vi "Launch Nested Actor with Map.vi"(8 "error in (no error)":errorcluster, 11 "Calling Actor in":refnum<class "Calling Actor.lvclass">) -> (0 "error out":errorcluster, 3 "Calling Actor out":refnum<class "Calling Actor.lvclass">)   [LabVIEW 2019, in "Calling Actor.lvlib" / "Calling Actor.lvclass"]
uses:
  Calling Actor.lvclass
  C:/Program Files (x86)/National Instruments/LabVIEW 2019/vi.lib/ActorFramework/Actor/Actor.lvclass
  Nested Actor/Nested Actor.lvclass
  Calling Actor.lvclass/Calling Actor.ctl
  <vilib>/ActorFramework/Actor/Actor.lvclass
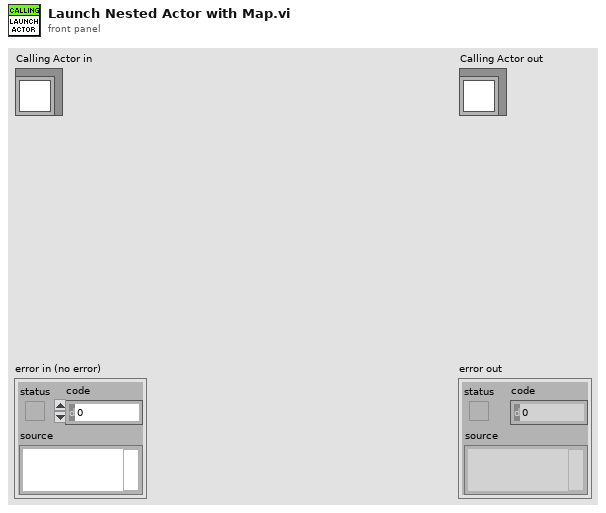
[diagram p1: front panel]
types:
  T1 = map{string, refnum<class "Message Enqueuer.lvclass">}
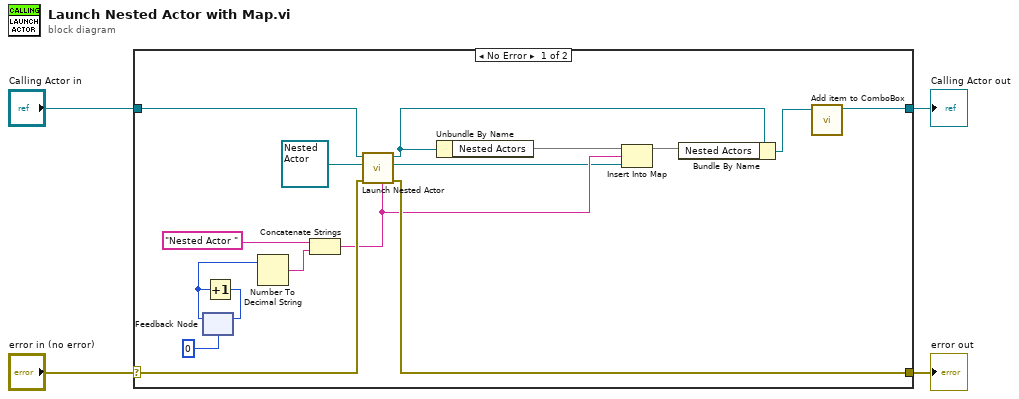
[diagram p0: block diagram]
diagram:
  n1 = case shown="No Error" "error in (no error)" {
    selector: "error in (no error)" -> [w19 w22]
    tunnel: [w18 w22] -> w3
    tunnel: [w11 w21] -> w1
    tunnel: "Calling Actor in" -> [w20 w21]
    frame No Error {
      n2 = feedback #1(0) -> (w14:i32)
      n3 = Increment(x=w14) -> (x+1=w15:i32)
      n4 = feedback-in #1(w15) -> ()
      n5 = Number To Decimal String(number=w14) -> (decimal integer string=w13:string)  [unwired: 1 in]
      n6 = Concatenate Strings("Nested Actor ", w13) -> (w9:string)
      n7 = call <vilib>:"Launch Nested Actor.vi"("Debug Alias"=w9, "error in (no error)"=w19, "Nested Actor"=refnum<class "Nested Actor.lvclass"> refnum ("Nested Actor.lvlib:Nested Actor.lvclass"), "Caller Actor in"=w20) -> ("error out"=w18:errorcluster, "Nested Actor's Enqueuer"=w8:refnum<class "Message Enqueuer.lvclass">, "Caller Actor out"=w7:refnum<class "Calling Actor.lvclass">)  [unwired: 5 in]
      n8 = Unbundle By Name(w7) -> ("Nested Actors"=w10:T1)
      n9 = Insert Into Map(map in=w10, key=w9, value=w8) -> (map out=w5:T1)  [unwired: 2 out]
      n10 = Bundle By Name(cluster=w7, "Nested Actors"=w5) -> (w6:refnum<class "Calling Actor.lvclass">)
      n11 = call "Add item to ComboBox.vi"("Calling Actor in"=w6) -> ("Calling Actor out"=w11:refnum<class "Calling Actor.lvclass">)  [unwired: 9 in, 1 out]
    }
    frame Error {
    }
  }
  "error out" <- w3
  "Calling Actor out" <- w1
